vi "Labview_Calculator.vi"() -> ()   [LabVIEW 2015]
panel:
  in  "ClearHist":bool
  in  "Array 2":string[](array[string])
  out "Array":string[](array[string])
  out "Numeric":i32
  in  "stop":bool
  out "Label.Text":string
  out "current time":timestamp format="%<%X\n%x>T"
  in  "CE":bool
  in  "C":bool
  in  "=":bool
  in  "Sqrt":bool
  in  "1/x":bool
  in  "backspace":bool
  in  "+/-":bool
  in  "/":bool
  in  "*":bool
  in  "-":bool
  in  "+":bool
  in  ".":bool
  in  "3":bool
  in  "6":bool
  in  "9":bool
  in  "8":bool
  in  "5":bool
  in  "2":bool
  in  "0":bool
  in  "7":bool
  in  "4":bool
  in  "1":bool
  # "Calculator"
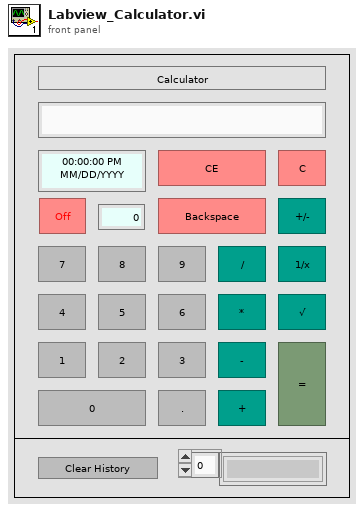
[diagram p1: front panel]
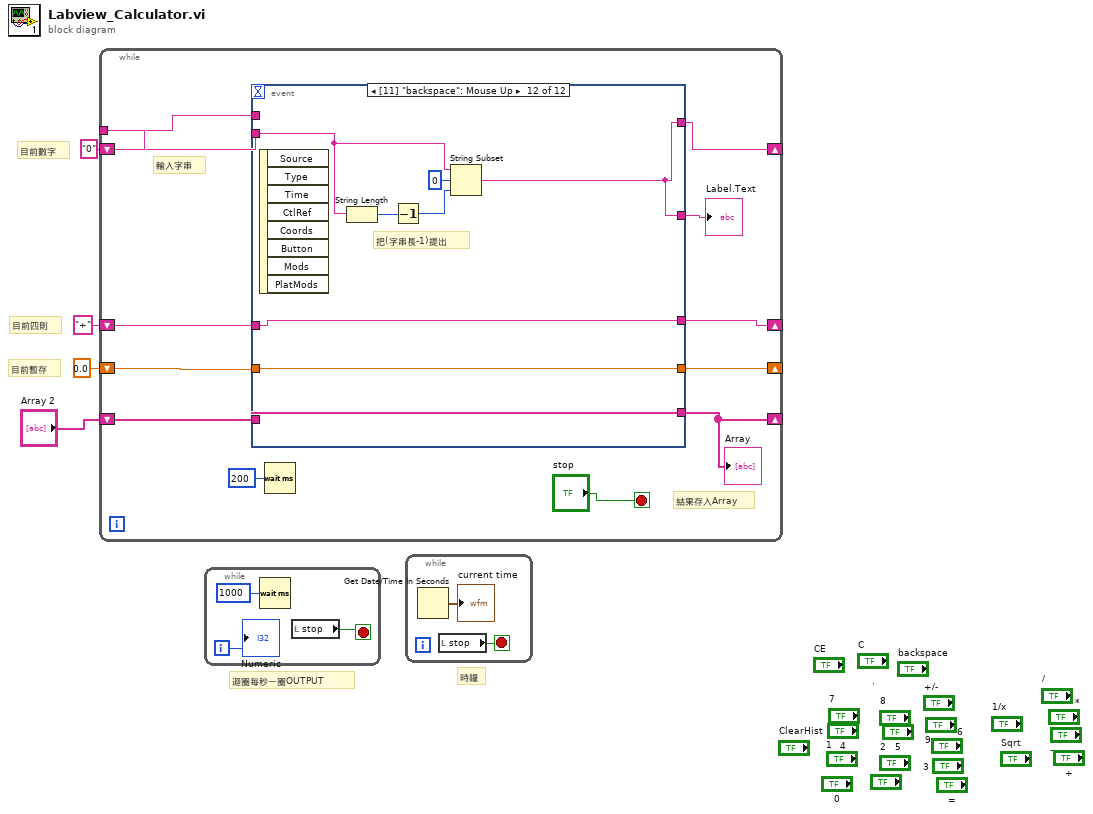
[diagram p0: block diagram]
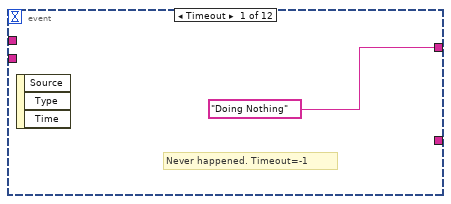
[diagram p2: hidden frame]
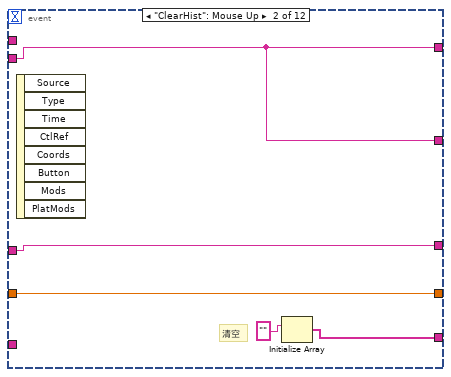
[diagram p3: hidden frame]
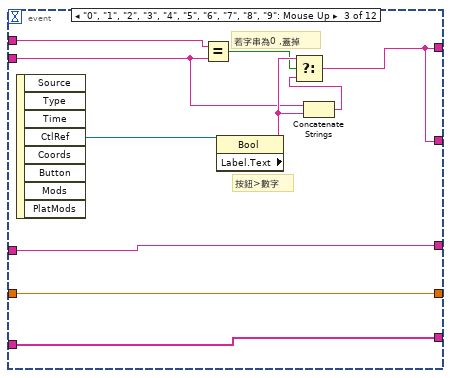
[diagram p4: hidden frame]
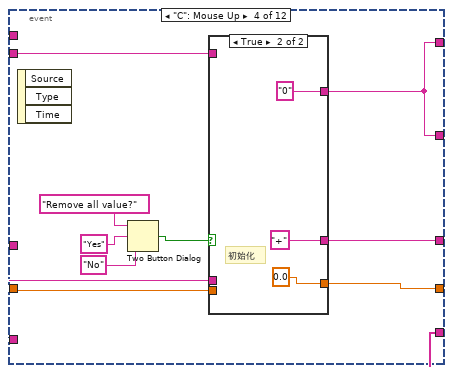
[diagram p5: hidden frame]
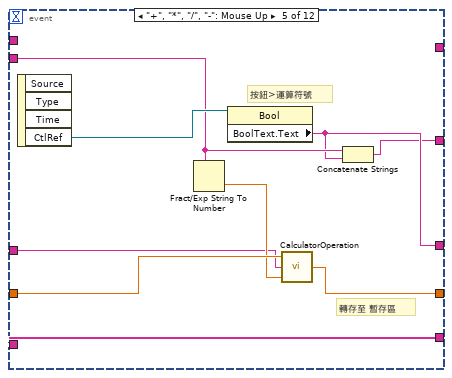
[diagram p7: hidden frame]
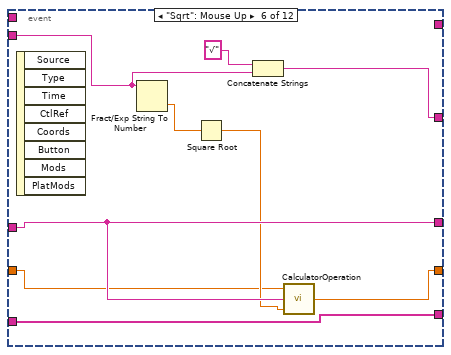
[diagram p8: hidden frame]
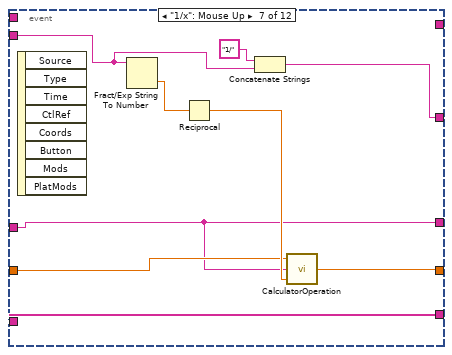
[diagram p9: hidden frame]
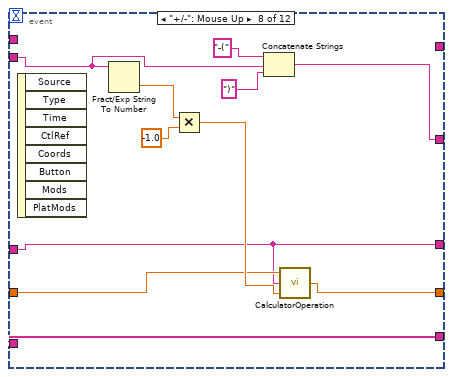
[diagram p10: hidden frame]
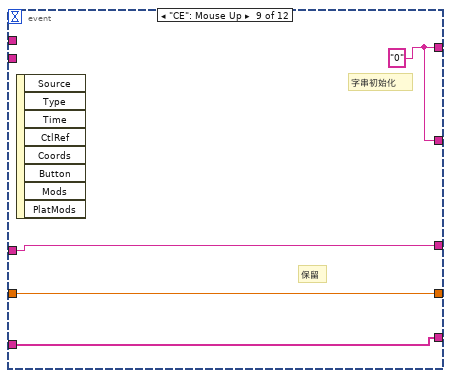
[diagram p11: hidden frame]
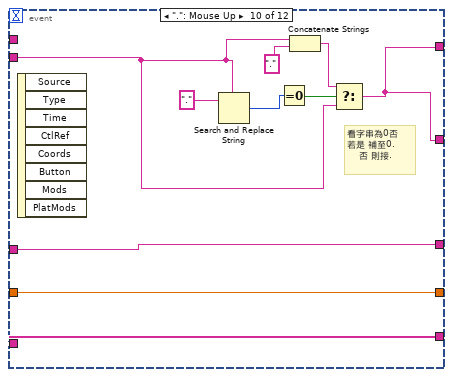
[diagram p12: hidden frame]
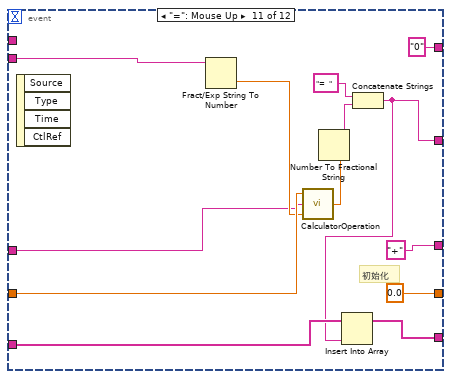
[diagram p13: hidden frame]
diagram:
  w4 = "0"
  # "目前數字"
  # "時鐘"
  # "迴圈每秒一圈OUTPUT"
  # "目前暫存"
  # "目前四則"
  n1 = while {
    shift-right: [w8] -> _
    shift-left: w4 -> [w16]
    tunnel: w4 -> [w15]
    shift-right: [w11] -> _
    shift-left: "+" -> [w13]
    shift-right: [w12] -> _
    shift-left: 0.0 -> [w10]
    shift-right: [w6] -> _
    shift-left: "Array 2" -> [w5]
    stop <- "stop" stop-if-true
    # "結果存入Array"
    # "輸入字串"
    n2 = event shown="[11] \"backspace\": Mouse Up" {
      selector: _ -> [_ _ _ _ _ _ _ _ _ _ _ _]
      dyn-events: _ -> [_ _ _ _ _ _ _ _ _ _ _ _]
      timeout: _ -> [_ _ _ _ _ _ _ _ _ _ _ _]
      tunnel: w16 -> [_ w19 w28 w34 w53 w61 w71 w81 _ w96 w114 w122]
      tunnel: ["Doing Nothing" w19 w24 w37 _ _ _ _ w89 w93 "0" ("Label.Text") w116] -> w8
      tunnel: w15 -> [_ _ w29 _ _ _ _ _ _ _ _ _]
      tunnel: w10 -> [_ w21 w25 w35 w58 w63 w74 w84 w91 w94 w113 w117]
      tunnel: w13 -> [_ w20 w26 w36 w56 w66 w73 w83 w90 w95 w111 w118]
      tunnel: [_ w21 w25 w38 w55 w65 w72 w82 w91 w94 0.0 w117] -> w12
      tunnel: [_ w20 w26 w39 w52 w66 w73 w83 w90 w95 "+" w118] -> w11
      tunnel: [_ w19 w24 w37 w51 w60 w69 w78 w89 w93 w103 w116] -> w7
      tunnel: w5 -> [_ _ w23 w33 w50 w59 w68 w77 w88 w92 w104 w115]
      tunnel: [_ w18 w23 w33 w50 w59 w68 w77 w88 w92 w102 w115] -> w6
      event Timeout {
        # "Never happened. Timeout=-1"
        n3 = event-data() -> ()  [unwired: 1 in, 3 out]
      }
      event "ClearHist": Mouse Up {
        # "清空"
        n4 = event-data() -> ()  [unwired: 1 in, 8 out]
        n5 = Initialize Array("") -> (w18:string[])  [unwired: 1 in]
      }
      event "0", "1", "2", "3", "4", "5", "6", "7", "8", "9": Mouse Up {
        # "若字串為0 ,蓋掉"
        # "按鈕>數字"
        n6 = event-data() -> ("CtlRef"=w32:refnum<vi>)  [unwired: 1 in, 7 out]
        n7 = Equal?(x=w29, y=w28) -> (x = y?=w27:bool)
        n8 = property class="Bool"(reference=w32) -> ("Label.Text"=w30:string)  [unwired: 1 in, 2 out]
        n9 = Concatenate Strings(w28, w30) -> (w31:string)
        n10 = Select(t=w30, s=w27, f=w31) -> (s? t:f=w24:string)
      }
      event "C": Mouse Up {
        n11 = event-data() -> ()  [unwired: 1 in, 3 out]
        n12 = Two Button Dialog(message="Remove all value?", 1:"No" ("F button name (\"Cancel\")"), 2:"Yes" ("T button name (\"OK\")")) -> (T button?=w40:bool)
        n13 = case shown="True" w40 {
          tunnel: [w46 "+"] -> w39
          tunnel: [w45 0.0] -> w38
          tunnel: [w44 "0"] -> w37
          tunnel: w36 -> [w46 _]
          tunnel: w35 -> [w45 _]
          tunnel: w34 -> [w44 _]
          frame False {
          }
          frame True {
            # "初始化"
          }
        }
      }
      event "+", "*", "/", "-": Mouse Up {
        # "轉存至 暫存區"
        # "按鈕>運算符號"
        n14 = event-data() -> ("CtlRef"=w54:refnum<vi>)  [unwired: 1 in, 3 out]
        n15 = Fract/Exp String To Number(string=w53) -> (number=w57:dbl)  [unwired: 3 in, 1 out]
        n16 = property class="Bool"(reference=w54) -> ("BoolText.Text"=w52:string)  [unwired: 1 in, 2 out]
        n17 = call "CalculatorOperation.vi"("Numeric 2"=w57, "String"=w56, "Numeric"=w58) -> ("Numeric 3"=w55:dbl)
        n18 = Concatenate Strings(w53, w52) -> (w51:string)
      }
      event "Sqrt": Mouse Up {
        n19 = event-data() -> ()  [unwired: 1 in, 8 out]
        n20 = Fract/Exp String To Number(string=w61) -> (number=w67:dbl)  [unwired: 3 in, 1 out]
        n21 = Square Root(x=w67) -> (sqrt(x)=w64:dbl)
        n22 = Concatenate Strings("√", w61) -> (w60:string)
        n23 = call "CalculatorOperation.vi"("Numeric 2"=w64, "String"=w66, "Numeric"=w63) -> ("Numeric 3"=w65:dbl)
      }
      event "1/x": Mouse Up {
        n24 = event-data() -> ()  [unwired: 1 in, 8 out]
        n25 = Fract/Exp String To Number(string=w71) -> (number=w76:dbl)  [unwired: 3 in, 1 out]
        n26 = Reciprocal(x=w76) -> (1/x=w75:dbl)
        n27 = Concatenate Strings("1/", w71) -> (w69:string)
        n28 = call "CalculatorOperation.vi"("Numeric 2"=w75, "String"=w73, "Numeric"=w74) -> ("Numeric 3"=w72:dbl)
      }
      event "+/-": Mouse Up {
        n29 = event-data() -> ()  [unwired: 1 in, 8 out]
        n30 = Fract/Exp String To Number(string=w81) -> (number=w86:dbl)  [unwired: 3 in, 1 out]
        n31 = Multiply(x=w86, y=-1.0) -> (x*y=w85:dbl)
        n32 = Concatenate Strings("-(", w81, ")") -> (w78:string)
        n33 = call "CalculatorOperation.vi"("Numeric 2"=w85, "String"=w83, "Numeric"=w84) -> ("Numeric 3"=w82:dbl)
      }
      event "CE": Mouse Up {
        w89 = "0"
        # "字串初始化"
        # "保留"
        n34 = event-data() -> ()  [unwired: 1 in, 8 out]
      }
      event ".": Mouse Up {
        # "看字串為0否\n若是 補至0.\n    否 則接."
        n35 = event-data() -> ()  [unwired: 1 in, 8 out]
        n36 = Search and Replace String(input string=w96, search string="." ("replace string (\"\")")) -> (number of replacements=w101:i32)  [unwired: 6 in, 3 out]
        n37 = Equal To 0?(x=w101) -> (x = 0?=w100:bool)
        n38 = Concatenate Strings(w96, ".") -> (w99:string)
        n39 = Select(t=w99, s=w100, f=w96) -> (s? t:f=w93:string)
      }
      event "=": Mouse Up {
        # "初始化"
        n40 = event-data() -> ()  [unwired: 1 in, 4 out]
        n41 = Fract/Exp String To Number(string=w114) -> (number=w112:dbl)  [unwired: 3 in, 1 out]
        n42 = call "CalculatorOperation.vi"("Numeric 2"=w112, "String"=w111, "Numeric"=w113) -> ("Numeric 3"=w110:dbl)
        n43 = Number To Fractional String(number=w110) -> (F-format string=w106:string)  [unwired: 3 in]
        n44 = Concatenate Strings("=  ", w106) -> (w103:string)
        n45 = Insert Into Array(array=w104, new element=w103) -> (w102:string[])  [unwired: 1 in]
      }
      event "backspace": Mouse Up {
        # "把(字串長-1)提出"
        n46 = event-data() -> ()  [unwired: 1 in, 8 out]
        n47 = String Length(string=w122) -> (length=w120:i32)
        n48 = Decrement(x=w120) -> (x-1=w119:i32)
        n49 = String Subset(string=w122, offset (0)=0, length (rest)=w119) -> (substring=w116:string)
      }
    }
    "Label.Text" <- w7
    "Array" <- w6
    n50 = Wait (ms)(milliseconds to wait=u32 200) -> ()  [unwired: 1 out]
  }
  n51 = while {
    i -> [w124]
    stop <- w123 stop-if-true
    n52 = Wait (ms)(milliseconds to wait=u32 1000) -> ()  [unwired: 1 out]
    n53 = local read "stop"() -> (w123:bool)
    "Numeric" <- w124
  }
  n54 = while {
    stop <- w126 stop-if-true
    n55 = Get Date/Time In Seconds() -> (seconds since 1Jan1904=→"current time":timestamp)
    n56 = local read "stop"() -> (w126:bool)
  }
